vi "Initialize.vi"(8 "error in":errorcluster, 10 "Application Directory":path) -> (0 "error out":errorcluster, 3 "SLL out":refnum<class "SLL.lvclass">)   [LabVIEW 2023, in "SLL.lvlib" / "SLL.lvclass"]
uses:
  SLL.lvclass
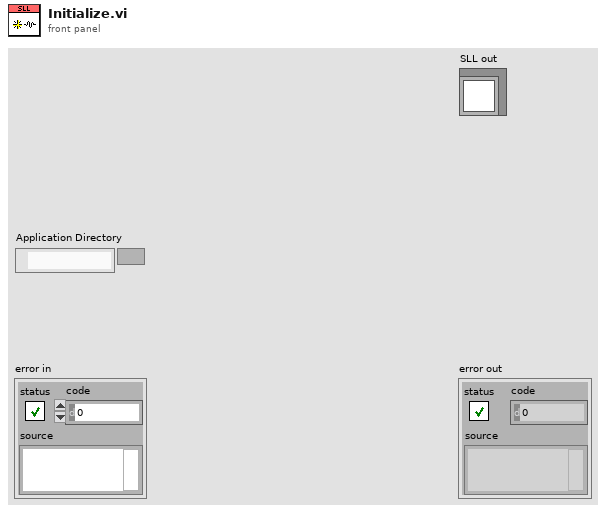
[diagram p1: front panel]
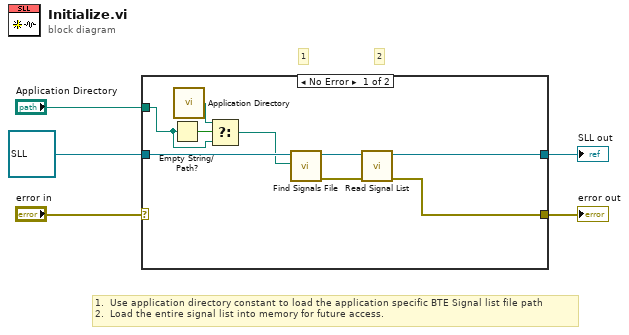
[diagram p0: block diagram]
diagram:
  # "1.  Use application directory constant to load the application specific BTE Signal list file path\n2.  Load the entire signal list into memory for future access."
  # "2"
  # "1"
  n1 = case shown="No Error" "error in" {
    selector: "error in" -> [_ w16]
    tunnel: [w10 w16] -> w4
    tunnel: [w11 w15] -> w1
    tunnel: refnum<class "SLL.lvclass"> refnum ("Signal List Loader in") -> [w14 w15]
    tunnel: "Application Directory" -> [w7 _]
    frame No Error {
      n2 = Empty String/Path?(string/path=w7) -> (empty?=w9:bool)
      n3 = call <vilib>:"Application Directory.vi"() -> ("Application Directory"=w8:path)
      n4 = Select(t=w8, s=w9, f=w7) -> (s? t:f=w6:path)
      n5 = call "Find Signals File.vi"("Application Directory"=w6, "SLL in"=w14) -> ("error out"=w12:errorcluster, "SLL out"=w13:refnum<class "SLL.lvclass">)  [unwired: 8 in]
      n6 = call "Read Signal List.vi"("error in"=w12, "SLL in"=w13) -> ("error out"=w10:errorcluster, "SLL out"=w11:refnum<class "SLL.lvclass">)  [unwired: 8 in]
    }
    frame Error {
    }
  }
  "error out" <- w4
  "SLL out" <- w1
